vi "Approximate Polygon (Douglas-Peucker).vi"(7 "Is Closed? (Default: True)":bool=TRUE, 8 "error in (no error)":errorcluster, 10 "Epsilon":dbl=0.001 format="%#_13g", 11 "Points in":T1[](array[typedef])) -> (0 "error out":errorcluster, 3 "Points out":T1[](array[typedef]))   [LabVIEW 2020, in "g_ar_toolkit.shape.lvlib"]
uses:
  g_ar_toolkit.shape.lvlib
  g_ar_toolkit.common/Image Point (Integer).ctl
  g_ar_toolkit.common/g_ar_toolkit.common.lvlib
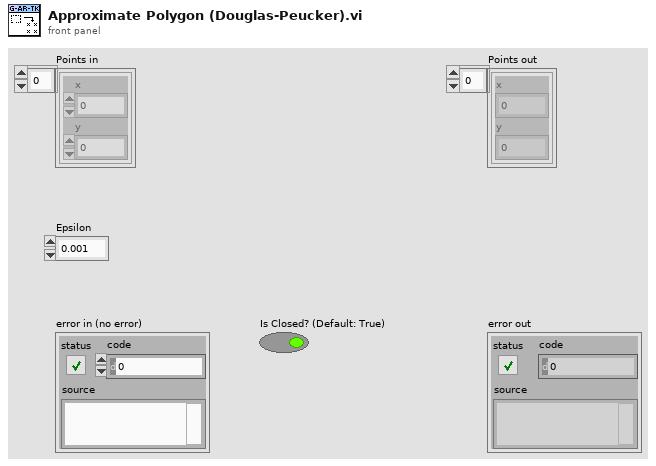
[diagram p1: front panel]
types:
  T1 = typedef "g_ar_toolkit.common.lvlib/Image Point (Integer).ctl" = cluster{"x":i32, "y":i32}
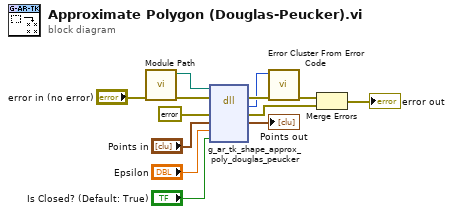
[diagram p0: block diagram]
diagram:
  n1 = call "Module Path.vi"("error in (no error)"="error in (no error)") -> ("error out"=w2:errorcluster, "Path"=w1:path)  [unwired: 9 in]
  n2 = dll-call lib="?" fn="g_ar_tk_shape_approx_poly_douglas_peucker" ("g_ar_toolkit.*.*:g_ar_tk_image_draw_line")(path in=w1, error in=w2, "error_cluster"=errorcluster {"status"=FALSE, "code"=0, "source"=""} ("error constant"), "points"="Points in", "epsilon"="Epsilon", "is_closed"="Is Closed? (Default: True)") -> (error out=w11:errorcluster, "MgErr"=w10:i32, "error_cluster"=w7:errorcluster, "points"=→"Points out":T1[])  [unwired: 3 in, 1 out]
  n3 = call <vilib>:"Error Cluster From Error Code.vi"("error in (no error)"=w11, "error code (0)"=w10) -> ("error out"=w9:errorcluster)  [unwired: 7 in]
  n4 = Merge Errors(w9, w7) -> (→"error out":errorcluster)
